vi "Line squaring.vi"(11 "NXT/EV3":T1) -> (3 "NXT/EV3":T1)   [LabVIEW 2016]
uses:
  <vilib>/NXT/Subs/LVHSConnector.ctl
  <vilib>/NXT/LegoClasses/BrickReference/BrickReference.lvclass
  Lining.ctl
  <vilib>/NXT/Block Support/NXT_OutputPort.ctl
  <vilib>/NXT/Block Support/NXT_InputPort.ctl
  <vilib>/NXT/NXTIO Xnodes/NXTIONodeSubVIs/NXTStopMotors.vi
  <vilib>/NXT/Dual Mode Library/Sensors/EV3_Color_Reflect.vi
  <vilib>/NXT/NXTIO Xnodes/NXTIONodeSubVIs/NXTMoveMotors.vi
  <vilib>/NXT/NXTIO Xnodes/NXTIOXNode/NXTIO.xnode
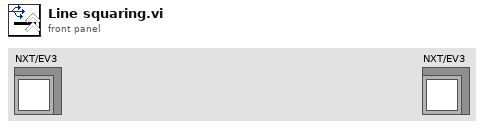
[diagram p1: front panel]
types:
  T1 = typedef "LVHSConnector.ctl" = refnum<class "BrickReference.lvclass">
  T2 = typedef "NXT_OutputPort.ctl" = u8
  T3 = typedef "Lining.ctl" = enum16{"Color readings", "Motor switch", "Lined", "Stop"}
  T4 = typedef "NXT_InputPort.ctl" = u32
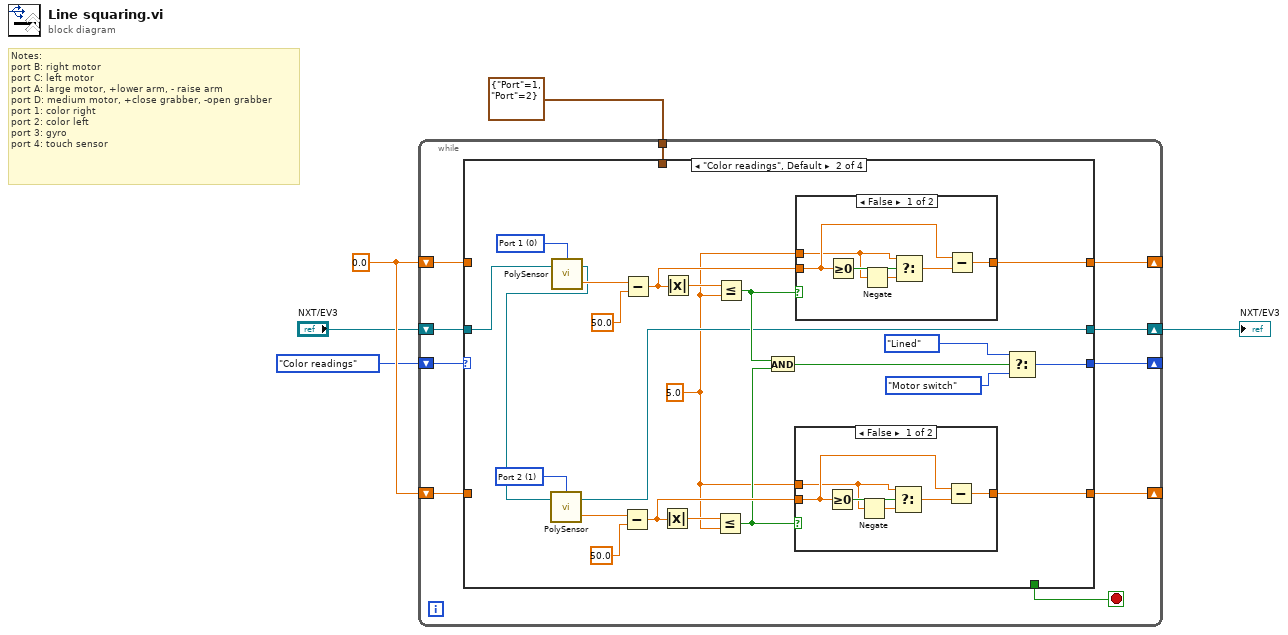
[diagram p0: block diagram]
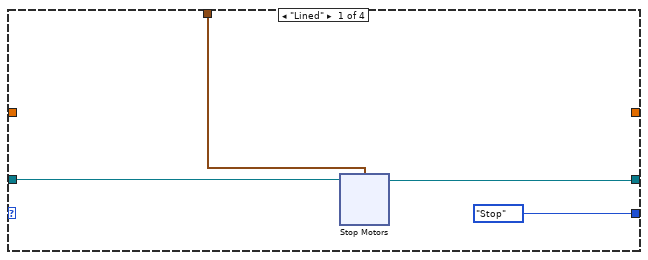
[diagram p2: hidden frame]
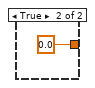
[diagram p3: hidden frame]
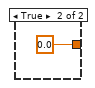
[diagram p4: hidden frame]
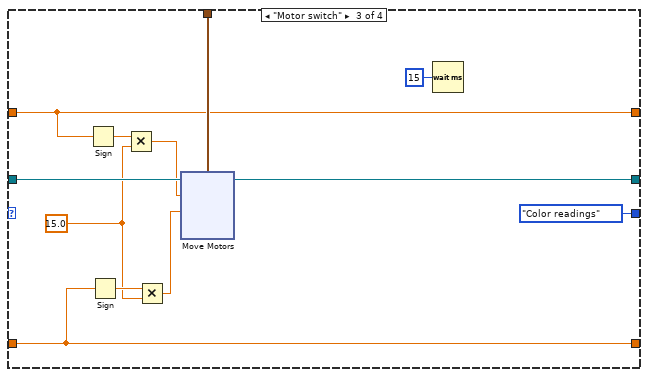
[diagram p5: hidden frame]
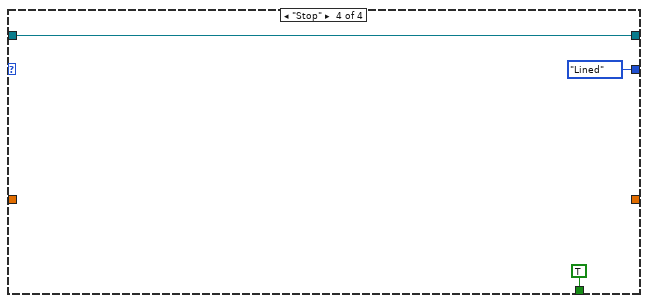
[diagram p6: hidden frame]
diagram:
  w5 = 0.0
  # "Notes:\nport B: right motor\nport C: left motor\nport A: large motor, +lower arm, - raise arm \nport D: medium motor, +close grabber, -open grabber\nport 1: color right\nport 2: color left\nport 3: gyro\nport 4: touch sensor"
  n1 = while {
    shift-right: [w12] -> _
    shift-left: Lining."Color readings" ("Enum") -> [w15]
    shift-right: [w14] -> _
    shift-left: w5 -> [w11]
    shift-right: [w13] -> _
    shift-left: w5 -> [w10]
    shift-right: [w9] -> w1
    shift-left: "NXT/EV3" -> [w8]
    tunnel: cluster{"Port":T2, "Port":T2} {"Port"=1, "Port"=2} ("Motor") -> [w6]
    stop <- w7 stop-if-true
    n2 = case shown="\"Color readings\", Default" w15 {
      tunnel: [_ w36 w70 _] -> w14
      tunnel: [_ w35 w66 _] -> w13
      tunnel: [Lining."Stop" ("Enum") w34 Lining."Color readings" ("Enum") Lining."Lined" ("Enum")] -> w12
      tunnel: w11 -> [_ _ w70 _]
      tunnel: w10 -> [_ _ w66 _]
      tunnel: [w18 w26 w64 w81] -> w9
      tunnel: w8 -> [w19 w28 w71 w81]
      tunnel: [_ _ _ TRUE] -> w7
      tunnel: w6 -> [w16 _ w72 _]
      frame "Lined" {
        n3 = xnode "Stop Motors"("Motors"=w16, "NXT/EV3"=w19) -> ("NXT/EV3"=w18:T1)
      }
      frame "Color readings", Default {
        w37 = T4 1 items=["Port 1", "Port 2", "Port 3", "Port 4"] ("Port (Port 1)")
        w25 = sgl 5.0 ("y")
        w46 = T4 0 items=["Port 1", "Port 2", "Port 3", "Port 4"] ("Port (Port 1)")
        n4 = call-poly <vilib>:"PolySensor.vi"("NXT/EV3"=w28, "Port (Port 1)"=w46) -> ("Scaled Value"=w45:sgl, "NXT/EV3"=w27:T1)  [unwired: 1 in]
        n5 = call-poly <vilib>:"PolySensor.vi"("NXT/EV3"=w27, "Port (Port 1)"=w37) -> ("Scaled Value"=w38:sgl, "NXT/EV3"=w26:T1)  [unwired: 1 in]
        n6 = Subtract(x=w38, y=sgl 50.0) -> (x-y=w41:sgl)
        n7 = Subtract(x=w45, y=sgl 50.0) -> (x-y=w42:sgl)
        n8 = Absolute Value(x=w41) -> (abs(x)=w40:sgl)
        n9 = Absolute Value(x=w42) -> (abs(x)=w43:sgl)
        n10 = Less Or Equal?(x=w40, y=w25) -> (x <= y?=w31:bool)
        n11 = Less Or Equal?(x=w43, y=w25) -> (x <= y?=w32:bool)
        n12 = And(x=w32, y=w31) -> (x .and. y?=w30:bool)
        n13 = case shown="False" w31 {
          tunnel: w41 -> [w50 _]
          tunnel: [w49 0.0] -> w35
          tunnel: w25 -> [w47 _]
          frame False {
            n14 = Greater Or Equal To 0?(x=w50) -> (x >= 0?=w52:bool)
            n15 = Negate(x=w47) -> (-x=w48:sgl)
            n16 = Select(t=w47, s=w52, f=w48) -> (s? t:f=w51:sgl)
            n17 = Subtract(x=w50, y=w51) -> (x-y=w49:sgl)
          }
          frame True {
          }
        }
        n18 = case shown="False" w32 {
          tunnel: w42 -> [w57 _]
          tunnel: [w56 0.0] -> w36
          tunnel: w25 -> [w54 _]
          frame False {
            n19 = Greater Or Equal To 0?(x=w57) -> (x >= 0?=w59:bool)
            n20 = Negate(x=w54) -> (-x=w55:sgl)
            n21 = Select(t=w54, s=w59, f=w55) -> (s? t:f=w58:sgl)
            n22 = Subtract(x=w57, y=w58) -> (x-y=w56:sgl)
          }
          frame True {
          }
        }
        n23 = Select(t=Lining."Lined" ("Enum"), s=w30, f=Lining."Motor switch" ("Enum")) -> (s? t:f=w34:T3)
      }
      frame "Motor switch" {
        w61 = 15.0 ("y")
        n24 = Sign(1:w70) -> (0:w69:dbl)
        n25 = Sign(1:w66) -> (0:w67:dbl)
        n26 = Multiply(x=w69, y=w61) -> (x*y=w68:dbl)
        n27 = Multiply(x=w67, y=w61) -> (x*y=w65:dbl)
        n28 = xnode "Move Motors"("Power/Speed 2"=w65, "Power/Speed 1"=w68, "Motors"=w72, "NXT/EV3"=w71) -> ("NXT/EV3"=w64:T1)
        n29 = Wait (ms)(milliseconds to wait=u32 15) -> ()  [unwired: 1 out]
      }
      frame "Stop" {
      }
    }
  }
  "NXT/EV3" <- w1
